vi "Gen model.vi"(6 "Interharm Cycles":dbl format="%.2f", 7 "V Coeff":dbl[](array[numeric]), 8 "Samples":i32=256, 9 "Fund Cycles":dbl=5.0 format="%.2f", 10 "Ramp in Model?":bool, 11 "No. Harmonics":i32=3) -> (1 "Ave Fund dCyc":dbl format="%.8e", 2 "Fund Cyc out":dbl format="%.8f", 3 "Model":dbl[][](array[numeric])=[[0.8700000000000001, 0.20875056464296693], [0.9249826350988861, 0.4505035907525611], [0.9718736897302015, 0.5750353163272757], [1.0030127595647964, 0.8298668876185543], [1.0121122630042265, 1.032133519853725], [0.995032669206001, 1.104735711760241], [0.9502318355094973, 1.2833196512252172], [0.8788385832147048, 1.2744477770756046], [0.7843551085476521, 1.3248298237807001], [0.6720456325166916, 1.3457395768681155], [0.5481123945563754, 1.2523700294813285], [0.4187885854059658, 1.3041455347894606], [0.2894871812929066, 1.3136533912801827], [0.1641337046067148, 1.145071180816352], [0.04478140671405345, 1.0023706886685475], [-0.06843640224198161, 0.9512922769701945], [-0.17701379293464392, 0.901170307998975], [-0.2834883681870865, 0.7647632304052223], [-0.39065993987772896, 0.7510585389342208], [-0.5007367381342565, 0.6305354156634336], [-0.6145470910168083, 0.4633925450016063], [-0.730947194944489, 0.4247159192911491], [-0.8465289242841515, 0.32519750698396904], [-0.9556892650346911, 0.4242675007814095], [-1.0510708245915188, 0.2685805072819846], [-1.1243283230719925, 0.28047028573076876], [-1.1671267707375539, 0.11326005862737727], [-1.172240252133262, 0.0506049057026155], [-1.134601255935653, -0.03752594369534071], [-1.0521522428747574, -0.0370158652767865], [-0.9263736863689529, -0.1413326535128248], [-0.7624033009901501, -0.17949192027476404], [-0.5687142167775155, -0.3050644297025635], [-0.3563782948264474, -0.34608990762742936], [-0.13799663674002444, -0.5018150490187354], [0.07357506300769859, -0.5713700195671704], [0.2665496589490305, -0.6593492212766714], [0.4314151809552584, -0.7187575896341312], [0.5618735296332487, -0.8024188507126513], [0.6553936411277644, -0.9084380722566848], [0.713311072954646, -0.8984996622860263], [0.7404646086395309, -0.8968609137090725], [0.7444203332562479, -0.9322777762367387], [0.7343866429772116, -0.8855863755219832], [0.7199627072384246, -0.7848040288220445], [0.7098828031691764, -0.7606077253619594], [0.7109171123690592, -0.6480101953796419], [0.7270664033690102, -0.47815374108214637], [0.7591468189497723, -0.2645147481023593], [0.8048074879057162, -0.028432350412204346], [0.8589652701049623, 0.19812145556998761], [0.9145856239916719, 0.3751571532917678], [0.9636938707939111, 0.5820953921242241], [0.9984730104085984, 0.7876150383584607], [1.0122963684301343, 0.887089274442824], [1.0005565364821116, 1.1616065888288951], [0.961184194026963, 1.1865553635396815], [0.8947967374012649, 1.2612201866124244], [0.8044705179474078, 1.2612455917541745], [0.6951842352595714, 1.3137017770412782], [0.5730270551039177, 1.2726269187617438], [0.4442968817967142, 1.2017190608177217], [0.31462751486600965, 1.2730026618947967], [0.18827641896286645, 1.15847058190871], [0.06767868540529937, 1.0188252680395502], [-0.04666866471115491, 0.9999658943564707], [-0.15597855334306054, 0.9172324275496434], [-0.2626409703814945, 0.8667905907420775], [-0.36947126155523635, 0.8405606945003923], [-0.47885979877215024, 0.702661202680202], [-0.5919600092468957, 0.6067492353425383], [-0.7080484132208208, 0.5391364195172218], [-0.8241672365303432, 0.41482870956397006], [-0.9351204718371973, 0.3468827931438487], [-1.0338434965319048, 0.2837260574119542], [-1.1121116676639418, 0.19860508409737856], [-1.1615024710436619, 0.07268786813090256], [-1.174486092931505, 0.11573719261279843], [-1.1454964938407355, 0.017397679077799585], [-1.0718326540090728, -0.11956241948364507], [-0.9542582624542976, -0.09416649766869271], [-0.7972054374852668, -0.22718209580750176], [-0.6085391676041872, -0.28517527508916096], [-0.3988971599008292, -0.27999794166544817], [-0.1806767764813522, -0.4293801456926952], [0.03321109718906248, -0.4954577071567689], [0.23066874031602821, -0.6262073853090656], [0.40165373628138856, -0.5888117729156264], [0.5391807930485207, -0.7617671788593521], [0.6399575977551826, -0.740288089706312], [0.704575991685528, -0.8820362156064765], [0.7372372117636857, -0.9390572577926327], [0.7450502074977225, -0.8398869379127274], [0.7369970002564002, -0.9576441211358697], [0.7227013255536706, -0.8669190247541692], [0.7111607486787834, -0.7266311670438899], [0.7096049393592365, -0.600660070398808], [0.7226236352106015, -0.48392574833092306], [0.7516697709788472, -0.34488091735347876], [0.7949916179660154, -0.07725170367987387], [0.8479897033688216, 0.16142732009069977], [0.9039377303650447, 0.3145718726845918], [0.9549593921635237, 0.532462418990366], [0.9931212294875843, 0.7632432725802332], [1.011489678922894, 0.9352503742621302], [1.0050095897772684, 1.0629490248572602], [0.9710901969752185, 1.191624835296949], [0.9098285654928095, 1.2473823977336325], [0.8238535079076261, 1.3819785504287967], [0.7178273629648192, 1.3296149320128534], [0.597691118425531, 1.3598240331503386], [0.4697734204006876, 1.3155154307889068], [0.3399011771688781, 1.1957986138299408], [0.21264644543943262, 1.189295482683133], [0.09082166598926458, 1.0825153624980486], [-0.024703535619914563, 0.9773496280115861], [-0.13484017542894577, 0.9462645852783378], [-0.24180135184021556, 0.7850951156744397], [-0.3483848216736006, 0.7488660077525305], [-0.45713146101199037, 0.6667438234951946], [-0.5694948442145212, 0.6601689366402674], [-0.6851578520042456, 0.45537967102743515], [-0.801612846670605, 0.49095104265200984], [-0.9140851462715796, 0.3607780854765334], [-1.0158304091594912, 0.3110678841926792], [-1.0987820133565596, 0.32617302614632837], [-1.154472313340601, 0.09744523875826525], [-1.1751092482648366, 0.10200377460937352], [-1.1546633140451306, 0.15698634448569238], [-1.0898133631186575, -0.00485053324593919], [-0.980614268797077, -0.1149129203732361], [-0.8307834509835725, -0.23120450879640164], [-0.6475521514617899, -0.24351877579959405], [-0.44108459866472943, -0.3182456363908144], [-0.22352602729382606, -0.491742191177653], [-0.007790989199313134, -0.499374020240362], [0.19376046425849014, -0.47303134969846505], [0.3705943807855673, -0.7033169489623365], [0.5150629691189074, -0.7114717470372084], [0.6231200840887938, -0.8285226337234308], [0.6946031647935993, -0.8231276797061983], [0.7330486293605201, -0.9330826863267713], [0.7450680858164203, -0.9647559498133932], [0.7393693365979184, -0.8613279663870389], [0.7255514270684267, -0.8196781628035734], [0.7128308650141447, -0.7691022623643928], [0.7088629507274165, -0.7220023753356838], [0.7188071192866486, -0.5312797876012052], [0.744750502055605, -0.307884037869586], [0.7855544263167641, -0.15720426418612254], [0.8371311431639683, 0.07227903347538527], [0.893100594891199, 0.2763857351526654], [0.9457273401159718, 0.5181194561647154], [0.9870025482961208, 0.7295529725068781], [1.00971990073956, 0.9078241782995345], [1.0083992525190293, 1.046667495462454], [0.9799370376795555, 1.1481110251814675], [0.9239038711696007, 1.230178998896881], [0.8424616030271522, 1.3265354624519712], [0.7399268097675081, 1.361472154617459], [0.6220576128069546, 1.3655475235804715], [0.4951787825618921, 1.319657882449561], [0.36528102928208606, 1.2299948516375843], [0.23723136523390312, 1.1458288622253396], [0.11421246248082426, 1.0513854341764315], [-0.0025271228251685096, 0.9586456216930895], [-0.11357785823492837, 0.9158907573170648], [-0.2209480075608321, 0.858437261250843], [-0.3273849594059722, 0.7410248810741664], [-0.43554773998834745, 0.6880350203227756], [-0.5471634303328767, 0.6815864621331998], [-0.6623048799842509, 0.4768542952247339], [-0.7789115489574915, 0.5260948832118546], [-0.8926415888157597, 0.45176902414705844], [-0.9970960670751046, 0.3244956364876695], [-1.0844021738393421, 0.3825067562272959], [-1.1460889792926845, 0.1650814511706742], [-1.1741444416557905, 0.13084692159214414], [-1.162112385187981, 0.07947336298924873], [-1.106077527590621, 0.04704873578562869], [-1.005397112637538, -0.06799351891881242], [-0.8630681344140239, -0.05586793406643502], [-0.6856655658848854, -0.1925153349481452], [-0.4828432070125829, -0.29345529284730343], [-0.26644711687282285, -0.42438625007783537], [-0.04934410183934934, -0.49128655345593475], [0.1558928446454358, -0.5460422563802892], [0.33827940781077115, -0.6849589367866253], [0.4895330842859793, -0.745144280736345], [0.6048648396766387, -0.8493114326602984], [0.683350527581726, -0.8598696860499816], [0.7278375012358328, -0.9053979233711157], [0.7444019825686995, -0.9143382675645374], [0.7414307357898048, -0.895485526033128], [0.7284486292502996, -0.844562881336445], [0.7148453303059003, -0.8185485708224858], [0.7086654772704788, -0.6898954923409698], [0.7156158378173965, -0.5437278961762524], [0.7384118158622988, -0.3788774958365322], [0.7765385918171513, -0.19353536639804583], [0.826445704983225, 0.035325841260432186], [0.8821357826292254, 0.2861258033093544], [0.9360563224222337, 0.47213174941391217], [0.9801649460535071, 0.710076132442261], [1.0070184709724315, 0.8096020942345732], [1.0107370133400115, 1.0437798791789346], [0.9877157348361182, 1.1337026427699508], [0.9369955262394084, 1.2411880178657637], [0.8602542509044163, 1.376082887216869], [0.7614349423155644, 1.3035222114396967], [0.6460787916568994, 1.3548692756181941], [0.5204716343034841, 1.3602486754273464], [0.3907372530607346, 1.280308490052526], [0.2620158037402164, 1.1571734113161019], [0.137850479853791, 1.097198533628705], [0.019872482995765064, 0.9613386651248226], [-0.09217169527816652, 0.9632273813301749], [-0.20005905022774875, 0.921890369567652], [-0.30645437108818147, 0.7751910722961692], [-0.41410196950441114, 0.6937093656869546], [-0.5249742807152623, 0.5431548366284001], [-0.6395154239554076, 0.5886260768487407], [-0.7561061410904513, 0.46791782489342226], [-0.8708460787608004, 0.43456907979865583], [-0.9777043441952511, 0.3037878522598904], [-1.0690359586876568, 0.2386604366540441], [-1.1364077899416791, 0.1930787024058685], [-1.17163046729703, 0.12033917842633086], [-1.1678594585136837, 0.022103201368586747], [-1.1206138241147212, -0.010458301574682444], [-1.0285674999614367, -0.08434727390519992], [-0.8939947061387972, -0.12366664519477402], [-0.7227947996720571, -0.2588203283358907], [-0.5240767452711714, -0.29473156390567024], [-0.309341940697993, -0.40290511985314054], [-0.09135839595141335, -0.5110987662335421], [0.11713824500066443, -0.568869911016277], [0.3047565395246658, -0.6163940736487041], [0.4626100185634361, -0.6958359386999099], [0.5851811781266673, -0.8577671312812192], [0.670780646989338, -0.8551005833738381], [0.7215456203817554, -0.8838835597725312], [0.7429812460925722, -0.7858783513781383], [0.7431076930106021, -0.9337034335142879], [0.7313261826083914, -0.928483507692399], [0.71715254648668, -0.8395443208043323], [0.7089822058603388, -0.6969702688407385], [0.7130439004725946, -0.5758466163287059], [0.7326720647920522, -0.39962615765032694], [0.767983337106925, -0.27502728358479955], [0.815987465819832, 0.037579601659515655], [0.8711044561829376, 0.28504639194057846], [0.9260061702054447, 0.42310238192238603], [0.9726590199957142, 0.7488389174700572], [1.0034204254041956, 0.7751557777528282], [1.0120384061586543, 0.9634041766940674]] format="%.2f", 4 "Interharm Cyc out":dbl format="%_9f")   [LabVIEW 2014]
uses:
  <vilib>/Analysis/1siggen.llb/Ramp Pattern by Samples.vi
  <vilib>/Analysis/NI_AALBase.lvlib
panel:
  out "Model":dbl[][](graph)
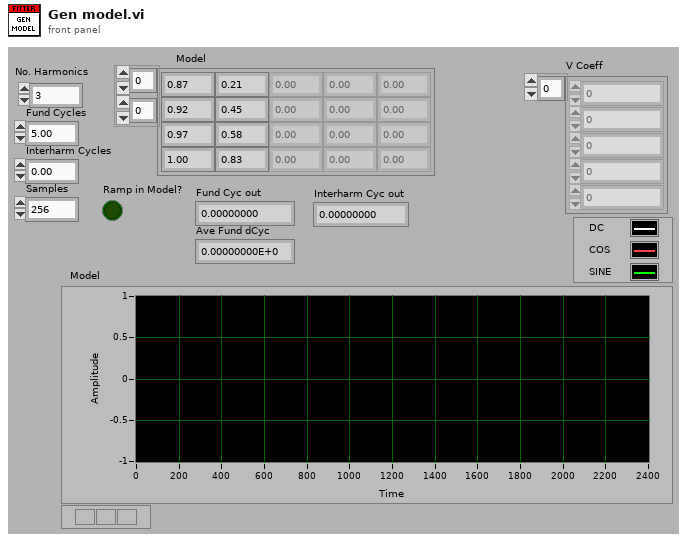
[diagram p1: front panel]
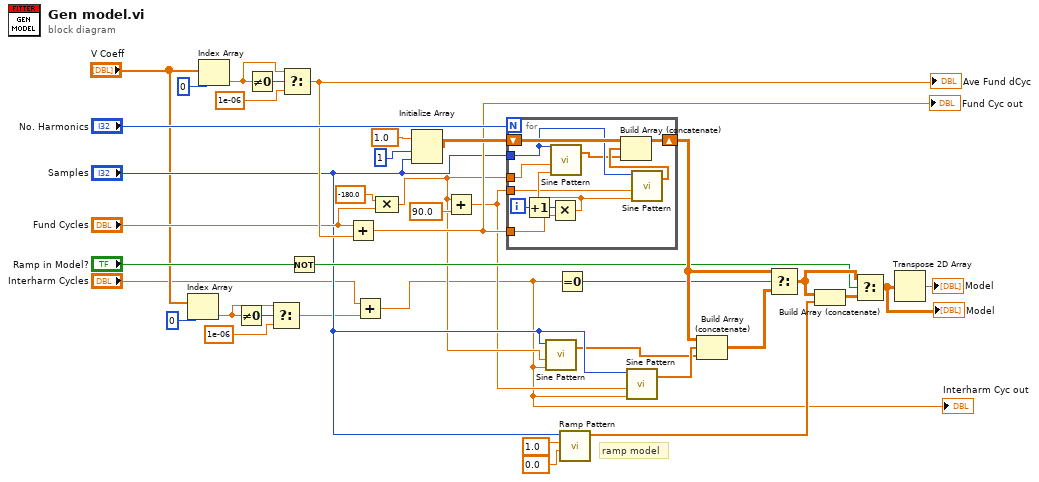
[diagram p0: block diagram]
diagram:
  # "ramp model"
  n1 = Index Array(array="V Coeff", index=0) -> (element=w8:dbl)
  n2 = Index Array(array="V Coeff", index=0) -> (element=w9:dbl)
  n3 = Not Equal To 0?(x=w8) -> (x != 0?=w6:bool)
  n4 = Not Equal To 0?(x=w9) -> (x != 0?=w28:bool)
  n5 = Select(t=w8, s=w6, f=1e-06) -> (s? t:f=w3:dbl)
  n6 = Select(t=w9, s=w28, f=1e-06) -> (s? t:f=w26:dbl)
  "Ave Fund dCyc" <- w26
  n7 = Not(x="Ramp in Model?") -> (.not. x?=w21:bool)
  n8 = Add(x="Fund Cycles", y=w26) -> (x+y=w34:dbl)
  "Fund Cyc out" <- w34
  n9 = Add(x="Interharm Cycles", y=w3) -> (x+y=w1:dbl)
  "Interharm Cyc out" <- w1
  n10 = Compound Arithmetic op=MULTIPLY(-180.0 ("y"), "Fund Cycles") -> (w12:dbl)
  n11 = Initialize Array(1.0 ("element"), 1 ("dimension size"), "Samples") -> (w37:dbl[][])
  n12 = Add(x=w12, y=90.0 ("phase(degrees)")) -> (x+y=w11:dbl)
  n13 = for {
    N: "No. Harmonics" -> [_]
    shift-right: [w48] -> w32
    shift-left: w37 -> [w47]
    tunnel: w34 -> [w46]
    tunnel: "Samples" -> [w43]
    tunnel: w12 -> [w42]
    tunnel: w11 -> [w39]
    i -> [w49]
    n14 = Increment(x=w49) -> (x+1=w45:i32)
    n15 = Multiply(x=w45, y=w46) -> (x*y=w44:dbl)
    n16 = call <vilib>:"Sine Pattern.vi"("cycles"=w44, "phase(degrees)"=w42, "samples"=w43) -> ("Sinusoidal Pattern"=w40:dbl[])  [unwired: 1 in, 1 out]
    n17 = call <vilib>:"Sine Pattern.vi"("cycles"=w44, "phase(degrees)"=w39, "samples"=w43) -> ("Sinusoidal Pattern"=w41:dbl[])  [unwired: 1 in, 1 out]
    n18 = Build Array (concatenate)(w47, w41, w40) -> (w48:dbl[][])
  }
  n19 = call <vilib>:"Sine Pattern.vi"("cycles"=w1, "phase(degrees)"=w12, "samples"="Samples") -> ("Sinusoidal Pattern"=w15:dbl[])  [unwired: 1 in, 1 out]
  n20 = Equal To 0?(x=w1) -> (x = 0?=w25:bool)
  n21 = call-poly <vilib>:"Ramp Pattern.vi"("start"=0.0, "end"=1.0, "samples"="Samples") -> ("Ramp Pattern"=w29:dbl[])  [unwired: 7 in, 1 out]
  n22 = call <vilib>:"Sine Pattern.vi"("cycles"=w1, "phase(degrees)"=w11, "samples"="Samples") -> ("Sinusoidal Pattern"=w16:dbl[])  [unwired: 1 in, 1 out]
  n23 = Build Array (concatenate)(w32, w16, w15) -> (w33:dbl[][])
  n24 = Select(t=w32, s=w25, f=w33) -> (s? t:f=w24:dbl[][])
  n25 = Build Array (concatenate)(w24, w29) -> (w23:dbl[][])
  n26 = Select(t=w24, s=w21, f=w23) -> (s? t:f=w19:dbl[][])
  "Model" <- w19
  n27 = Transpose 2D Array(2D array=w19) -> (transposed array=→"Model":dbl[][])
